vi "GLOBAL -Project MAIN.vi"() -> ()   [LabVIEW 2019]
uses:
  ctlProjMainSeqFNs.ctl
panel:
  out "EvntAuditAddr":refnum<user-event>
  in  "EvntPrjCntcts":refnum<user-event>
  in  "FNS":T1[](array[typedef])
  in  "CurrRowSiteMng":i32
  out "EXIT":bool
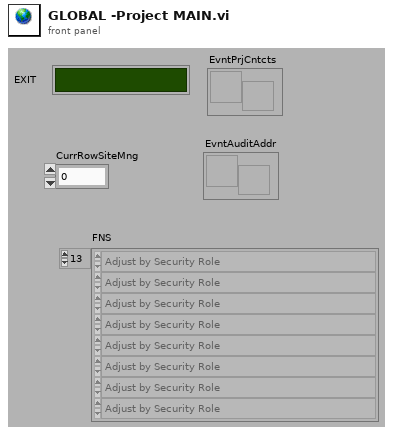
[diagram p1: front panel]
types:
  T1 = typedef "ctlProjMainSeqFNs.ctl" = enum16{"pre-init", "preinit01", "preinit02", "preinit03", "preinit04", "preinit05", "preinit06", "init", "idle", "Adjust by Security Role", "PULL -Project Info", "PULL -Companies", "PULL -Site Info", "PULL -Contacts", "PULL -Typical Cylinder Group", "BACK", "EDIT -Contact Internal or External", "ADD PROJECT -Register", "ADD PROJECT -Default Site", "ADD PROJECT -Default Field Density Folder and Site", "ADD PROJECT -Home Company and Contacts 00", "ADD PROJECT -Home Company and Contacts 01 ", "ADD PROJECT -Customer Company and Contacts", "ADD PROJECT -Test And Misc Costs", "ADD PROJECT -Add Typical Concrete Test Schedule", "EDIT PROJECT", "EDIT PROJECT -Test Cost", "EDIT PROJECT -Misc Cost", "EDIT -COMPANY DIV ID", "EDIT -COMPANY ROLE", "EDIT No Copy Suppliers", "EDIT Contact", "REFRESH -Main Grid Project List", "POPULATE -Starting Company and Contacs", "POPULATE -Company Contacts", "POPULATE -Home Contacts", "POPULATE -Existing Sites", "ADD Company Contact", "REMOVE PROJ CONTACT -External", "LOAD PROJECT -STEP 00", "LOAD PROJECT -STEP 01", "LOAD PROJECT -STEP 02", "UPDATE -Company IDX", "SHOW SELECTED CONTACT", "MISC POPULATE -Company", "MISC ARCHIVE COMPANY INFO", "DELETE -Company and Children", "CHECK CUSTOMER COMPANY", "HIGHLIGHT -1st Row", "MANAGE SITES", "LAUNCH -REPORT WINDOW", "RE-DO -Get Curr Contact Data", "RE-DO -Role & Company", "RE-DO -Contact ID and Send Mode", "GPS -Location Processing", "GPS -Audit Address", "GPS -Audit Post Processing", "error", "exit"}
diagram:
